vi "Acquire Start Stop Example.vi"() -> ()   [LabVIEW 2019]
uses:
  C:/Users/tim/Documents/kSAComm LabView Sample/kSACommInterface.dll
  kSACommInterface.dll
panel:
  out "Error":string
  out "Connected":bool
  in  "IP Address":string="192.168.0.169"
  in  "Exit":bool
  in  "Start/Stop Acquire":bool
  in  "Duration Type":i32(ring) items=["DURATION_TIME", "DURATION_DATA_POINTS", "DURATION_UNLIMITED"]
  in  "Run Name":string="LabVIEWTest"
  in  "Number of Samples":i16
  in  "Duration":dbl
  # "Upon starting this VI a connection will be made to a kSA application running on a PC using this IP address. The LED indicates successful connection."
  # "These are the parameters to be used during the \"Start Acquire\"."
  # "Press this button to \"Start\" or \"Stop\" the active acquire in the kSA application. The LED inside the button will indicate whether or not the Acquire is currently running."
  # "Press this button to cleanly disconnect from the kSA application and exit the VI"
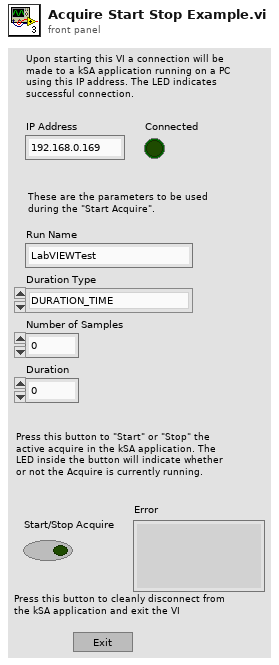
[diagram p1: front panel]
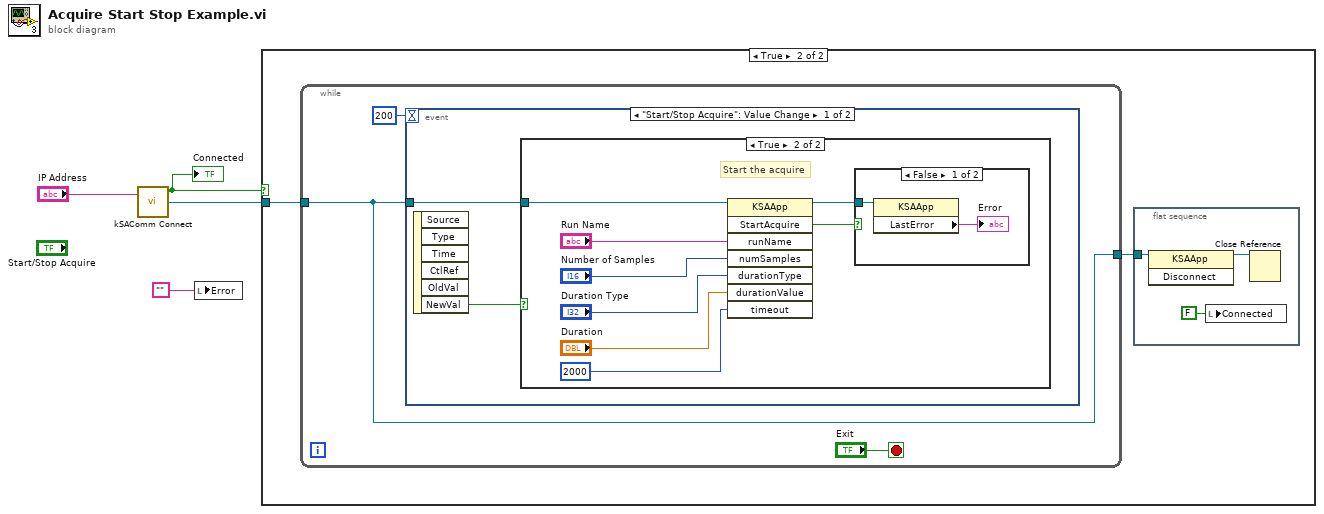
[diagram p0: block diagram]
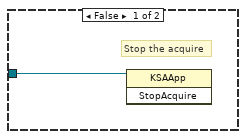
[diagram p3: hidden frame]
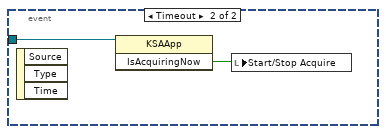
[diagram p5: hidden frame]
diagram:
  n1 = call "kSAComm Connect.vi"("IP Address"="IP Address") -> ("Connect"=w2:bool, "kSAComm ref out"=w3:refnum<k24>)  [unwired: 2 in]
  "Connected" <- w2
  n2 = local write "Error"("" ("Error")) -> ()
  n3 = case shown="True" w2 {
    tunnel: w3 -> [_ w6]
    frame False {
    }
    frame True {
      n4 = while {
        tunnel: w6 -> [w10]
        tunnel: [w10] -> w5
        stop <- "Exit" stop-if-true
        n5 = event shown="[0] \"Start/Stop Acquire\": Value Change" {
          selector: _ -> [_ _]
          dyn-events: _ -> [_ _]
          timeout: 200 -> [_ _]
          tunnel: w10 -> [w13 w27]
          event "Start/Stop Acquire": Value Change {
            n6 = event-data() -> ("NewVal"=w14:bool)  [unwired: 1 in, 5 out]
            n7 = case shown="True" w14 {
              tunnel: w13 -> [w15 w19]
              frame False {
                # "Stop the acquire"
                n8 = invoke class="KSAApp" method="StopAcquire"(reference=w15) -> ()  [unwired: 2 in, 3 out]
              }
              frame True {
                # "Start the acquire"
                n9 = invoke class="KSAApp" method="StartAcquire"(reference=w19, "runName"="Run Name", "numSamples"="Number of Samples", "durationType"="Duration Type", "durationValue"="Duration", "timeout"=2000) -> (reference out=w18:refnum<k24>, "StartAcquire"=w17:bool)  [unwired: 2 in, 6 out]
                n10 = case shown="False" w17 {
                  tunnel: w18 -> [w25 _]
                  frame False {
                    n11 = property class="KSAApp"(reference=w25) -> ("LastError"=→"Error":string)  [unwired: 1 in, 2 out]
                  }
                  frame True {
                  }
                }
              }
            }
          }
          event Timeout {
            n12 = event-data() -> ()  [unwired: 1 in, 3 out]
            n13 = invoke class="KSAApp" method="IsAcquiringNow"(reference=w27) -> ("IsAcquiringNow"=w26:bool)  [unwired: 2 in, 2 out]
            n14 = local write "Start/Stop Acquire"(w26) -> ()
          }
        }
      }
      n15 = flat-sequence {
        tunnel: w5 -> [w8]
        frame #0 {
          n16 = invoke class="KSAApp" method="Disconnect"(reference=w8) -> (reference out=w9:refnum<k24>)  [unwired: 2 in, 2 out]
          n17 = local write "Connected"(FALSE ("Connected")) -> ()
          n18 = Close Reference(reference=w9) -> ()  [unwired: 1 in, 1 out]
        }
      }
    }
  }
